vi "ERA_Build_Hankel.vi"(8 "error in (no error)":errorcluster, 11 "Measurements":dbl[][](array[numeric])) -> (0 "error out":errorcluster, 2 "H_1":T1, 3 "H_0":T1)   [LabVIEW 2017, in "AppPlugins.lvlib" / "EraPlugin.lvclass"]
uses:
  EraPlugin.lvclass
  <vilib>/Analysis/Matrix/Datatypes/RealMatrix.ctl
  <vilib>/Analysis/Matrix/Numeric/Conversions/Array To Matrix - RA2.vi
  <vilib>/Analysis/Matrix/NI_Matrix.lvlib
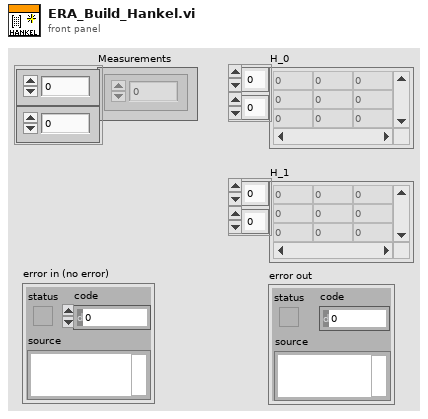
[diagram p1: front panel]
types:
  T1 = typedef "NI_Matrix.lvlib/RealMatrix.ctl" = dbl[][]
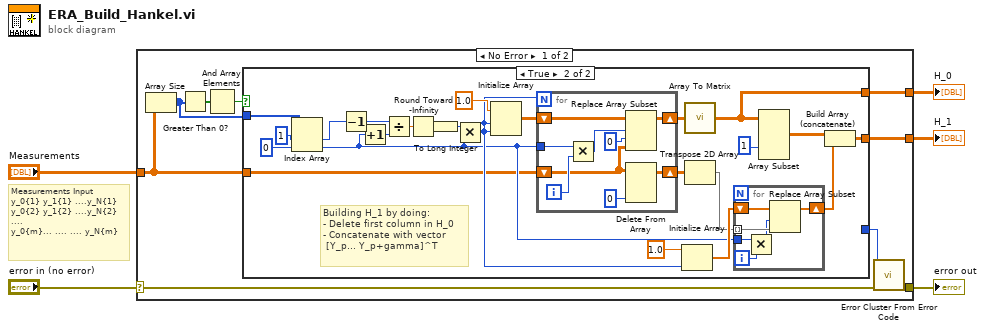
[diagram p0: block diagram]
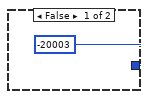
[diagram p2: hidden frame]
diagram:
  # "Measurements Input \ny_0{1} y_1{1} ....y_N{1}\ny_0{2} y_1{2} ....y_N{2}\n....\ny_0{m}... .... .... y_N{m}"
  n1 = case shown="No Error" "error in (no error)" {
    selector: "error in (no error)" -> [w7 w55]
    tunnel: "Measurements" -> [w14 _]
    tunnel: [w11 _] -> w4
    tunnel: [w10 _] -> w3
    tunnel: [w8 w55] -> w2
    frame No Error {
      n2 = Array Size(array=w14) -> (size(s)=w6:i32[])
      n3 = Greater Than 0?(x=w6) -> (x > 0?=w12:bool[])
      n4 = And Array Elements(Boolean array=w12) -> (logical AND=w13:bool)
      n5 = case shown="True" w13 {
        tunnel: [_ w28] -> w10
        tunnel: [_ w18] -> w11
        tunnel: w14 -> [_ w17]
        tunnel: [-20003 _] -> w9
        tunnel: w6 -> [_ w16]
        frame False {
        }
        frame True {
          # "Building H_1 by doing:\n- Delete first column in H_0\n- Concatenate with vector \n [Y_p... Y_p+gamma]^T"
          n6 = Index Array(array=w16, index #1=1 ("index"), index #2=0 ("index")) -> (element #1=w33:i32, element #2=w21:i32)
          n7 = Decrement(x=w33) -> (x-1=w32:i32)
          n8 = Increment(x=w21) -> (x+1=w30:i32)
          n9 = Divide(x=w32, y=w30) -> (x/y=w31:dbl)
          n10 = Round Toward -Infinity(1:w31) -> (0:w35:dbl)
          n11 = To Long Integer(number=w35) -> (32bit integer=w34:i32)
          n12 = Multiply(x=w34, y=w21) -> (x*y=w23:i32)
          n13 = Initialize Array(1.0 ("element"), w23, w23) -> (w37:dbl[][])
          n14 = for {
            N: w23 -> [_]
            shift-right: [w47] -> w29
            shift-left: w37 -> [w48]
            shift-right: [w53] -> w20
            shift-left: w17 -> [w46]
            tunnel: w21 -> [w50]
            i -> [w51]
            n15 = Multiply(x=w50, y=w51) -> (x*y=w49:i32)
            n16 = Replace Array Subset(array=w48, new element=w46, index (row)=w49, index (col)=0) -> (w47:dbl[][])
            n17 = Delete From Array(array=w46, index (col)=0 ("disabled index (col)")) -> (array with subset deleted=w53:dbl[][])  [unwired: 2 in, 1 out]
          }
          n18 = Initialize Array(1.0 ("element"), w23) -> (w25:dbl[])
          n19 = call-poly <vilib>:"Array To Matrix.vi"("Real 2D Array"=w29) -> ("Real Matrix"=w28:T1)
          n20 = Transpose 2D Array(2D array=w20) -> (transposed array=w19:dbl[][])
          n21 = for {
            tunnel: w19 -> [w43] mode=indexing
            shift-right: [w44] -> w22
            shift-left: w25 -> [w45]
            tunnel: w21 -> [w40]
            i -> [w42]
            n22 = Multiply(x=w40, y=w42) -> (x*y=w41:i32)
            n23 = Replace Array Subset(array=w45, new element=w43, index=w41) -> (w44:dbl[])
          }
          n24 = Array Subset(array=w28, index (col)=1 ("column 1")) -> (w26:T1)  [unwired: 3 in]
          n25 = Build Array (concatenate)(w26, w22) -> (w18:T1)
        }
      }
      n26 = call <vilib>:"Error Cluster From Error Code.vi"("error in (no error)"=w7, "error code (0)"=w9) -> ("error out"=w8:errorcluster)  [unwired: 7 in]
    }
    frame Error {
    }
  }
  "H_1" <- w4
  "H_0" <- w3
  "error out" <- w2
